vi "Test Request.vi"(8 "error in (no error)":errorcluster, 11 "Test Process Test in":refnum<class "Test Process Test.lvclass">) -> (0 "error out":errorcluster, 3 "Test Process Test out":refnum<class "Test Process Test.lvclass">)   [LabVIEW 2020, in "Test Process Test.lvclass"]
uses:
  Test Process Test.lvclass
  Test Process Test.lvclass/Test Process Test.ctl
  Test Process/Test Process.lvclass
  <vilib>/Astemes/Triarc Framework/Process/Process.lvclass
  C:/Program Files (x86)/National Instruments/LabVIEW 2020/vi.lib/Astemes/Triarc Framework/Process/Process.lvclass
  C:/Program Files (x86)/National Instruments/LabVIEW 2020/vi.lib/Astemes/Triarc Framework/Base/Base.lvclass
  C:/Program Files (x86)/National Instruments/LabVIEW 2020/vi.lib/Astemes/Triarc Framework/Error Handler Interface/Error Handler Interface.lvclass
  C:/Program Files (x86)/National Instruments/LabVIEW 2020/vi.lib/Astemes/Triarc Framework/Logging/Logging.lvclass
  C:/Users/anton/Documents/GitHub/triarc-debugger/test/Test Process/Test Process.lvclass
  <vilib>/Astemes/LUnit/Test Case.lvclass
  C:/Program Files (x86)/National Instruments/LabVIEW 2020/vi.lib/Astemes/Triarc Framework Test Suite/Process Test/Process Test.lvclass
  C:/Program Files (x86)/National Instruments/LabVIEW 2020/vi.lib/Astemes/Triarc Framework Test Suite/Base Class Test/Base Test.lvclass
  C:/Program Files (x86)/National Instruments/LabVIEW 2020/vi.lib/Astemes/LUnit/Test Case.lvclass
  C:/Users/anton/Documents/GitHub/triarc-debugger/test/Test Process Test/Test Process Test.lvclass
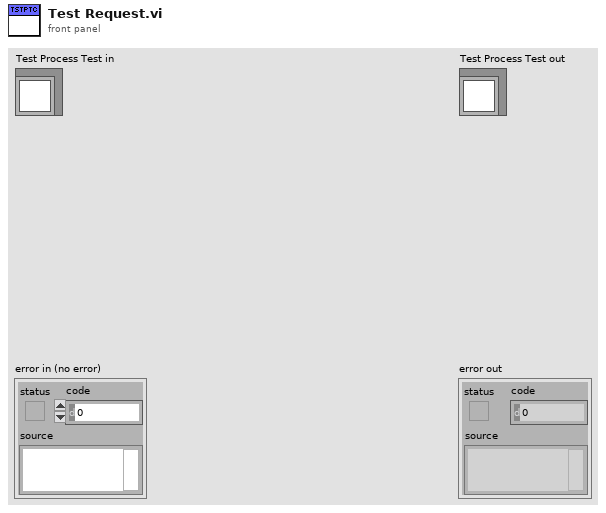
[diagram p1: front panel]
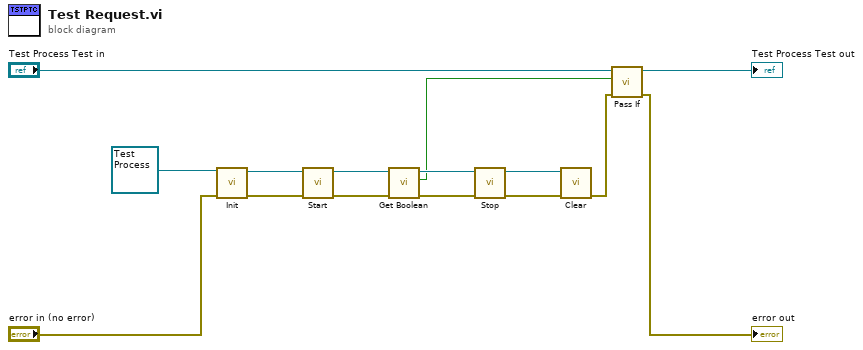
[diagram p0: block diagram]
diagram:
  n1 = call-dynamic "Init.vi"("error in (no error)"="error in (no error)", "Process In"=refnum<class "Test Process.lvclass"> refnum ("Test Process.lvclass")) -> ("error out"=w13:errorcluster, "Process Out"=w14:refnum<class "Test Process.lvclass">)  [unwired: 8 in]
  n2 = call <vilib>:"Start.vi"("error in (no error)"=w13, "Process In"=w14) -> ("error out"=w12:errorcluster, "Process Out"=w6:refnum<class "Test Process.lvclass">)  [unwired: 7 in, 1 out]
  n3 = call "Get Boolean.vi"("error in (no error)"=w12, "Test Process In"=w6) -> ("error out"=w10:errorcluster, "Boolean"=w4:bool, "Test Process Out"=w11:refnum<class "Test Process.lvclass">)  [unwired: 7 in]
  n4 = call <vilib>:"Stop.vi"("error in (no error)"=w10, "Process In"=w11) -> ("error out"=w8:errorcluster, "Process Out"=w9:refnum<class "Test Process.lvclass">)  [unwired: 7 in, 1 out]
  n5 = call-dynamic "Clear.vi"("error in (no error)"=w8, "Process In"=w9) -> ("error out"=w3:errorcluster)  [unwired: 9 in]
  n6 = call <vilib>:"Pass If.vi"("error in (no error)"=w3, "Pass?"=w4, "LUnit Test Case In"="Test Process Test in") -> ("error out"=→"error out":errorcluster, "LUnit Test Case Out"=→"Test Process Test out":refnum<class "Test Process Test.lvclass">)  [unwired: 7 in]
